vi "Datum_Image_Calibration.vi"(3 "Mode":T8=enum."Run VI", 5 "Traverse line In":T5={"Start X"=-1250.0, "Start Y"=-250.0, "Start Z"=180.0, "End X"=0.0, "End Y"=0.0, "End Z"=0.0, "No. of pts."=6, "Spacing"=enum."Linear", "Filename"=path "C:/Enflo_Data_Local/2015/EnFlo_Tunnel/Paul_Hayden/Calibrations/Cal_06-2015/Datum_Block_1.xls", "Tunnel Speed"=0.0, "Averaging time (min)"=0.01, "Extra Commands"="", "Carrier_1 Q (l/min)"=nan, "Carrier_2 Q (l/min)"=nan, "Trace Gas Concentration (%)"=nan, "Specific Arguments"="Datum_Image_Calibration.vi  ", "Comments"="", "Row No"=0, "Row Type Selector"=enum."Run VI Named:", "Completion time"="12:51  12-06-2015", "Row Duration (mins)"=0.11291999999999999, "No. of Valid pts."=6, "Meas Setup File"="Trav_Cam_Picture.xls"} {"Carrier_2 Q (l/min)" format="%#.2f"; "Row Duration (mins)" format="%#.1f"; "Row No" min=0; "Trace Gas Concentration (%)" min=0.0 format="%#_4f"; "Carrier_1 Q (l/min)" format="%#.2f"; "Tunnel Speed" format="%#.2f"; "Start X" format="%#.2f"; "Start Y" format="%#.2f"; "Start Z" format="%#.2f"; "End X" format="%#.2f"; "End Y" format="%#.2f"; "End Z" format="%#.2f"; "Averaging time (min)" min=0.0 format="%#.2f"}) -> (0 "Error Message":string, 1 "Status":T4, 2 "Traverse line Out":T5 {"Carrier_2 Q (l/min)" format="%#.2f"; "Row Duration (mins)" format="%#.1f"; "Row No" min=0; "Trace Gas Concentration (%)" min=0.0 format="%#_4f"; "Carrier_1 Q (l/min)" format="%#.2f"; "Tunnel Speed" format="%#.2f"; "Start X" format="%#.2f"; "Start Y" format="%#.2f"; "Start Z" format="%#.2f"; "End X" format="%#.2f"; "End Y" format="%#.2f"; "End Z" format="%#.2f"; "Averaging time (min)" min=0.0 format="%#.2f"})   [LabVIEW 2014]
uses:
  Gen Trav/Multi_Run_Status.ctl
  <vilib>/Analysis/NI_AALBase.lvlib
  <vilib>/Analysis/baseanly.llb/Mean (DBL).vi
  Utilities/Image acquisition and processing/Feature detection/Typedefs/Theta range.ctl
  Gen Trav/Spacing.ctl
  Gen Trav/Traverse_cluster.ctl
  Controls/User_Specific_mode.ctl
  Controls/Multi_run_mode.ctl
  <vilib>/userdefined/High Color/IMAQdx.ctl
  Utilities/Image acquisition and processing/Feature detection/Typedefs/ROI bounds.ctl
panel:
  in  "Theta range (deg)":T1={"theta max (deg)"=5.0, "theta min (deg)"=-5.0}
  in  "ROI to crop (pixels)":T2={"Xmax"=2147483647, "Ymax"=2147483647, "Xmin"=0, "Ymin"=160}
  out "Scale":dbl[](graph)
  out "Angle":dbl[](graph)
  out "Displacments":sgl[][](array[numeric])
  in  "Interface name":T3="cam2"
  in  "VideoMode":u32=9
  in  "Averaging time (s) (from end)":dbl=1.0
  in  "Duration (s)":dbl=10.0
  in  "FPS":u32=30
  in  "Video codec":string="Microsoft Video 1"
  # "X           Y            Z"
  # "Start"
  # "End"
  # "X           Y            Z"
  # "Start"
  # "End"
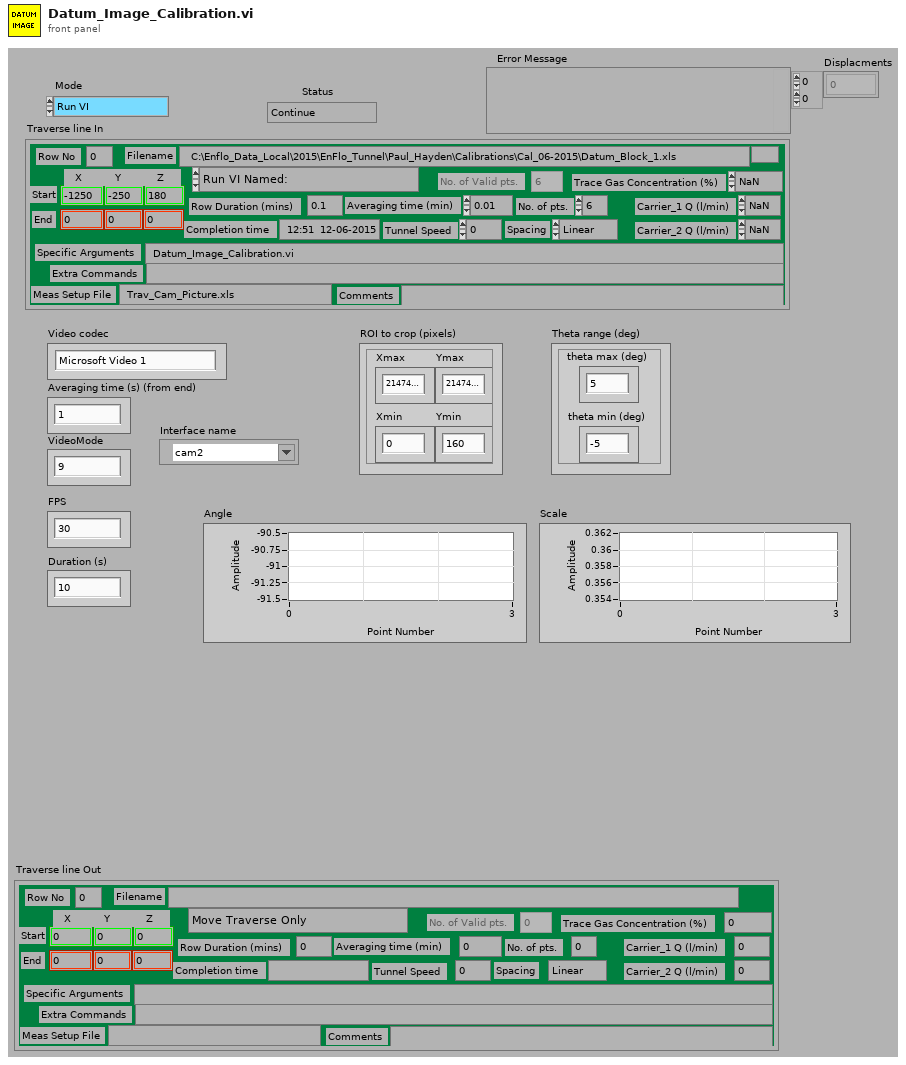
[diagram p1: front panel]
types:
  T1 = typedef "Theta range.ctl" = cluster{"theta max (deg)":dbl, "theta min (deg)":dbl}
  T2 = typedef "ROI bounds.ctl" = cluster{"Xmax":i32, "Ymax":i32, "Xmin":i32, "Ymin":i32}
  T3 = typedef "IMAQdx.ctl" = refnum<k21>
  T4 = typedef "Multi_Run_Status.ctl" = enum16{"Continue", "Jump to Next Point", "Jump to Next Row", "Jump To Fall Back", "Terminate Run"}
  T5 = typedef "Traverse_cluster.ctl" = cluster{"Start X":sgl, "Start Y":sgl, "Start Z":sgl, "End X":sgl, "End Y":sgl, "End Z":sgl, "No. of pts.":i32, "Spacing":T6, "Filename":path, "Tunnel Speed":dbl, "Averaging time (min)":dbl, "Extra Commands":string, "Carrier_1 Q (l/min)":dbl, "Carrier_2 Q (l/min)":dbl, "Trace Gas Concentration (%)":dbl, "Specific Arguments":string, "Comments":string, "Row No":i32, "Row Type Selector":T7, "Completion time":string, "Row Duration (mins)":dbl, "No. of Valid pts.":i32, "Meas Setup File":string}
  T6 = typedef "Spacing.ctl" = enum16{"Linear", "Log", "Gauss", "Specified", "N/A"}
  T7 = typedef "Multi_run_mode.ctl" = enum16{"Move Traverse Only", "Set Tunnel Speed Only", "Set Source Only", "Set Measurement Conditions", "Single Measurement", "Vertical Profile", "Lateral Profile", "Longitudinal Profile", "Explore Volume", "Multi-Axis Profile", "Auto Calibrate", "Meas Fast FID Bkgnd", "Check Beam Power", "Scanning Valve Measurement", "Run VI Named:", "Set ADAM Ch", "Wait (minutes)", "Send Message", "Synchronize With:", "Fall Back to this Row", "Turn Off Row Repeating", "Blank Row", "Traverse 3D Volume"}
  T8 = typedef "User_Specific_mode.ctl" = enum16{"Check VI only", "Run VI"}
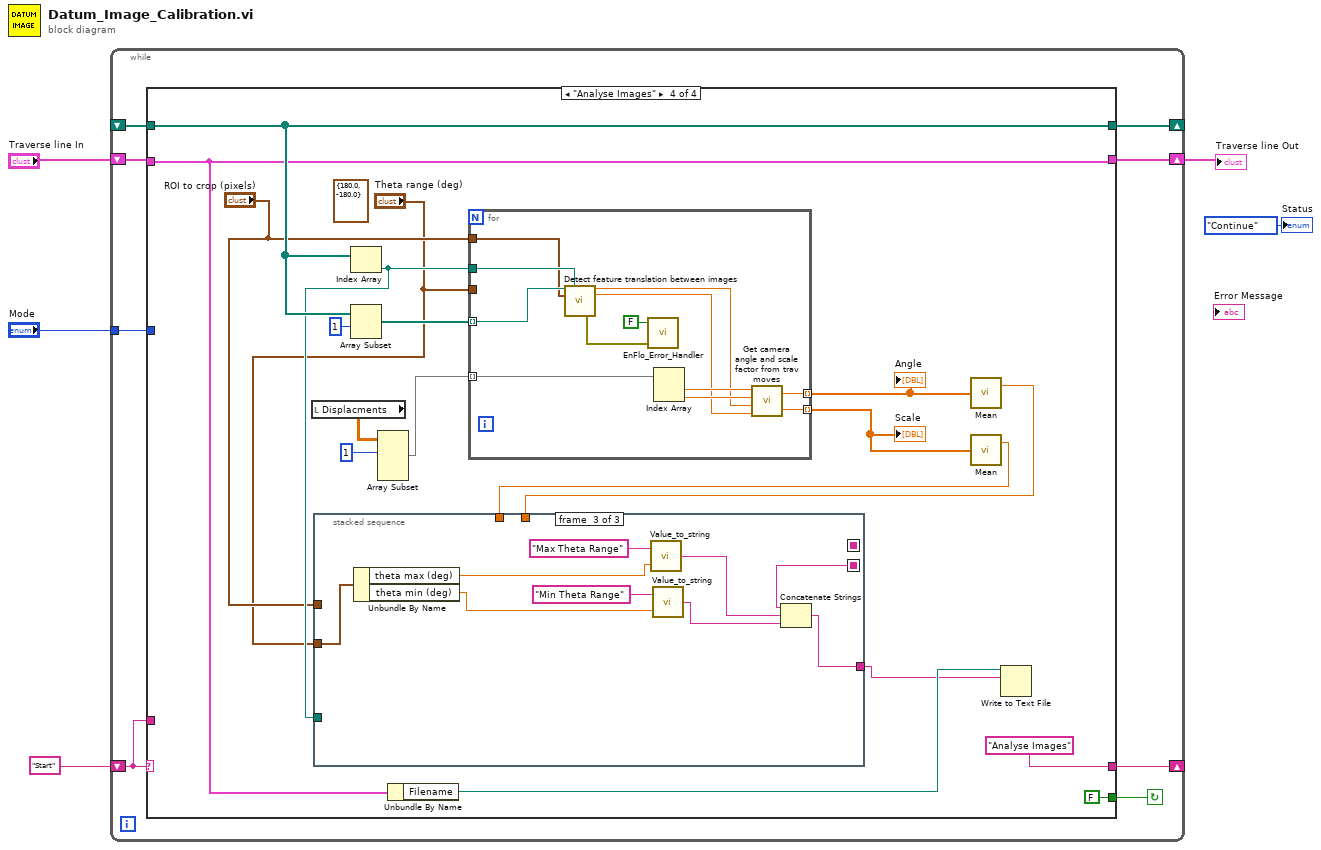
[diagram p0: block diagram]
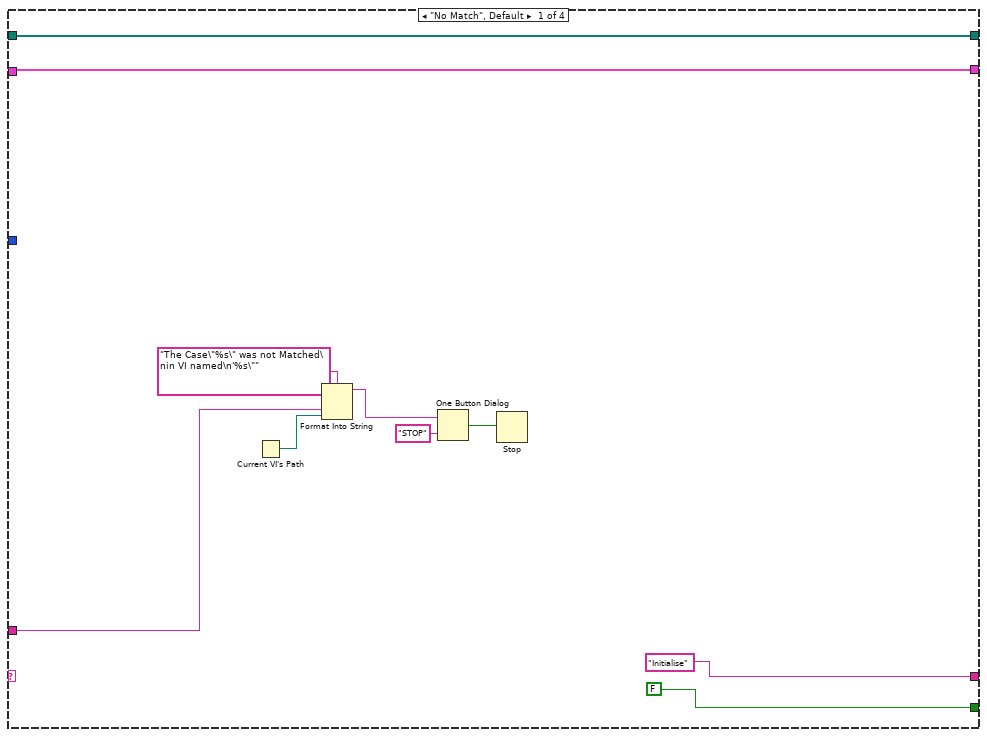
[diagram p2: hidden frame]
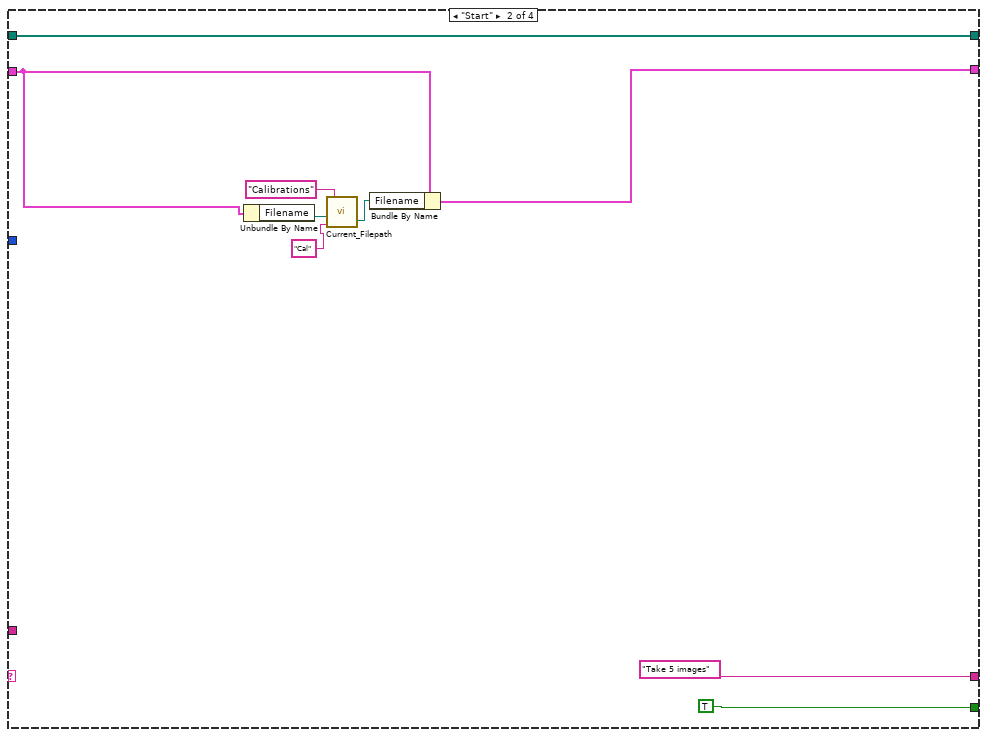
[diagram p3: hidden frame]
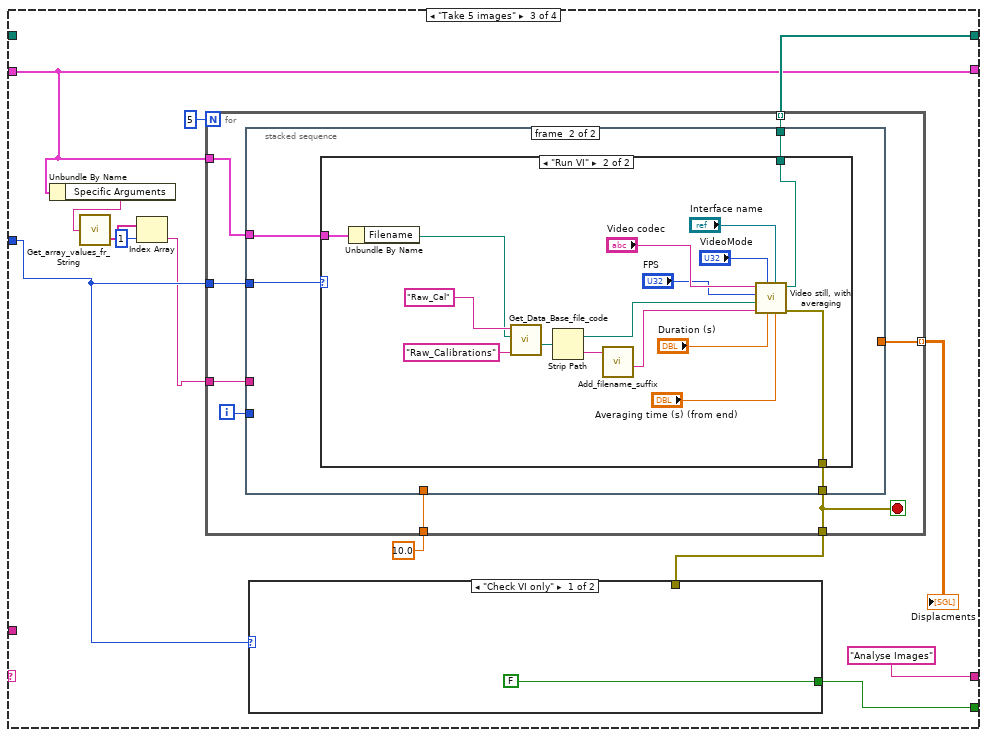
[diagram p4: hidden frame]
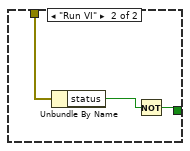
[diagram p5: hidden frame]
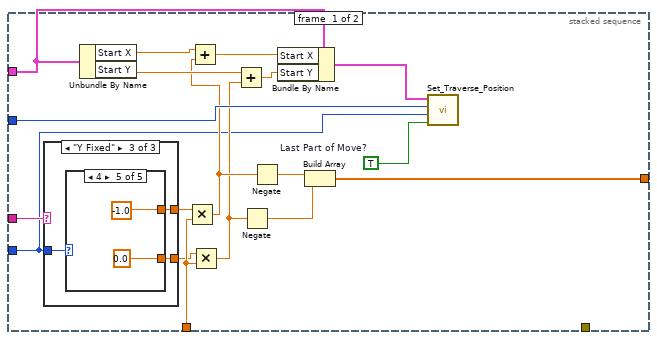
[diagram p6: hidden frame]
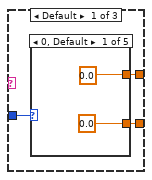
[diagram p7: hidden frame]
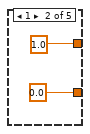
[diagram p8: hidden frame]
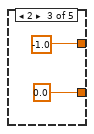
[diagram p9: hidden frame]
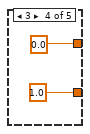
[diagram p10: hidden frame]
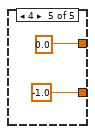
[diagram p11: hidden frame]
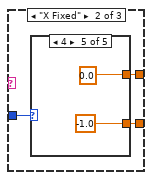
[diagram p12: hidden frame]
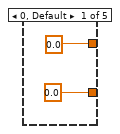
[diagram p13: hidden frame]
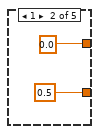
[diagram p14: hidden frame]
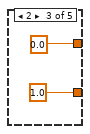
[diagram p15: hidden frame]
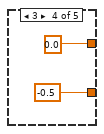
[diagram p16: hidden frame]
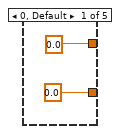
[diagram p17: hidden frame]
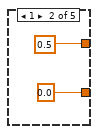
[diagram p18: hidden frame]
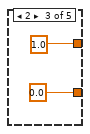
[diagram p19: hidden frame]
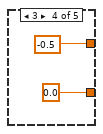
[diagram p20: hidden frame]
diagram:
  n1 = while {
    shift-left: "Start" -> [w11]
    shift-right: [w12] -> _
    tunnel: "Mode" -> [w10]
    shift-right: [w8] -> w1
    shift-left: "Traverse line In" -> [w9]
    shift-right: [w7] -> _
    shift-left: _ -> [w6]
    stop <- w13 continue-if-true
    n2 = case shown="\"Analyse Images\"" w11 {
      tunnel: [FALSE TRUE w40 FALSE] -> w13
      tunnel: ["Initialise" "Take 5 images" "Analyse Images" "Analyse Images"] -> w12
      tunnel: w11 -> [w18 _ _ _]
      tunnel: w10 -> [_ _ w41 _]
      tunnel: w9 -> [w15 w27 w37 w146]
      tunnel: [w15 w26 w37 w146] -> w8
      tunnel: [w14 w25 w42 w152] -> w7
      tunnel: w6 -> [w14 w25 _ w152]
      frame "No Match", Default {
        n3 = Current VI's Path() -> (path=w17:path)
        n4 = Format Into String(format string="The Case\"%s\" was not Matched\nin VI named\n'%s\"" ("Format String"), w18, w17) -> (resulting string=w21:string)  [unwired: 2 in, 1 out]
        n5 = One Button Dialog(message=w21, button name ("OK")="STOP") -> (true=w19:bool)
        n6 = Stop(stop? (T)=w19) -> ()
      }
      frame "Start" {
        n7 = Unbundle By Name(w27) -> ("Filename"=w29:path)
        n8 = call "Current_Filepath.vi"("Short_Name"="Cal" ("Data Type"), "Filename in"=w29, "Data Type"="Calibrations") -> ("Filename Out"=w24:path)  [unwired: 1 in, 1 out]
        n9 = Bundle By Name(cluster=w27, "Filename"=w24) -> (w26:T5)
      }
      frame "Take 5 images" {
        n10 = Unbundle By Name(w37) -> ("Specific Arguments"=w36:string)
        n11 = call "Get_array_values_fr_String.vi"("String Value"=w36) -> ("String array"=w35:string[])  [unwired: 1 out]
        n12 = Index Array(array=w35, index=1) -> (element=w33:string)
        n13 = for {
          N: 5 -> [_]
          tunnel: w37 -> [w57]
          tunnel: w41 -> [w56]
          tunnel: sgl 10.0 ("y") -> [w54]
          tunnel: [w53] -> w42 mode=indexing
          tunnel: [w52] -> w39
          tunnel: [w51] -> w38 mode=indexing
          tunnel: w33 -> [w50]
          i -> [w55]
          stop <- w52 stop-if-true
          n14 = stacked-sequence {
            tunnel: w57 -> [w67 w118]
            tunnel: w56 -> [w75 w117]
            tunnel: w55 -> [w59 _]
            tunnel: w54 -> [w72 _]
            tunnel: [_ w116] -> w53
            tunnel: [_ w115] -> w52
            tunnel: [w63 _] -> w51
            tunnel: w50 -> [w60 _]
            frame #0 {
              w58 = TRUE  # Last Part of Move?
              n15 = case shown="\"Y Fixed\"" w60 {
                tunnel: w59 -> [w78 w91 w104]
                tunnel: [w77 w90 w103] -> w73
                tunnel: [w76 w89 w102] -> w71
                frame Default {
                  n16 = case shown="0, Default" w78 {
                    tunnel: [sgl 0.0 ("Start Y") sgl 1.0 ("Start Y") sgl -1.0 ("Start Y") sgl 0.0 ("Start Y") sgl 0.0 ("Start Y")] -> w77
                    tunnel: [sgl 0.0 ("Start Y") sgl 0.0 ("Start Y") sgl 0.0 ("Start Y") sgl 1.0 ("Start Y") sgl -1.0 ("Start Y")] -> w76
                    frame 0, Default {
                    }
                    frame 1 {
                    }
                    frame 2 {
                    }
                    frame 3 {
                    }
                    frame 4 {
                    }
                  }
                }
                frame "X Fixed" {
                  n17 = case shown="4" w91 {
                    tunnel: [sgl 0.0 ("Start Y") sgl 0.0 ("Start Y") sgl 0.0 ("Start Y") sgl 0.0 ("Start Y") sgl 0.0 ("Start Y")] -> w90
                    tunnel: [sgl 0.0 ("Start Y") sgl 0.5 ("Start Y") sgl 1.0 ("Start Y") sgl -0.5 ("Start Y") sgl -1.0 ("Start Y")] -> w89
                    frame 0, Default {
                    }
                    frame 1 {
                    }
                    frame 2 {
                    }
                    frame 3 {
                    }
                    frame 4 {
                    }
                  }
                }
                frame "Y Fixed" {
                  n18 = case shown="4" w104 {
                    tunnel: [sgl 0.0 ("Start Y") sgl 0.5 ("Start Y") sgl 1.0 ("Start Y") sgl -0.5 ("Start Y") sgl -1.0 ("Start Y")] -> w103
                    tunnel: [sgl 0.0 ("Start Y") sgl 0.0 ("Start Y") sgl 0.0 ("Start Y") sgl 0.0 ("Start Y") sgl 0.0 ("Start Y")] -> w102
                    frame 0, Default {
                    }
                    frame 1 {
                    }
                    frame 2 {
                    }
                    frame 3 {
                    }
                    frame 4 {
                    }
                  }
                }
              }
              n19 = Unbundle By Name(w67) -> ("Start X"=w74:sgl, "Start Y"=w70:sgl)
              n20 = Multiply(x=w73, y=w72) -> (x*y=w65:sgl)
              n21 = Add(x=w74, y=w65) -> (x+y=w66:sgl)
              n22 = Multiply(x=w71, y=w72) -> (x*y=w64:sgl)
              n23 = Add(x=w70, y=w64) -> (x+y=w69:sgl)
              n24 = Negate(x=w64) -> (-x=w61:sgl)
              n25 = Negate(x=w65) -> (-x=w62:sgl)
              n26 = Bundle By Name(cluster=w67, "Start X"=w66, "Start Y"=w69) -> (w68:T5)
              n27 = Build Array(w62, w61) -> (w63:sgl[])
              n28 = call "Set_Traverse_Position.vi"("Last Part of Move?"=w58, "Currently on Point"=w59, "Simulate/Run"=w75, "Traverse line"=w68) -> ()  [unwired: 2 in, 1 out]
            }
            frame #1 {
              n29 = case shown="\"Run VI\"" w117 {
                tunnel: w118 -> [_ w128]
                tunnel: [path "" ("stripped path") w121] -> w116
                tunnel: [errorcluster {"status"=FALSE, "code"=0, "source"=""} ("Error Out") w123] -> w115
                frame "Check VI only" {
                }
                frame "Run VI" {
                  n30 = Unbundle By Name(w128) -> ("Filename"=w125:path)
                  n31 = call "Get_Data_Base_file_code.vi"("Data Type"="Raw_Calibrations", "Results Filename"=w125, "Short_Name"="Raw_Cal" ("Data Type")) -> ("Raw Data File Name"=w122:path)  [unwired: 1 in, 3 out]
                  n32 = Strip Path(path=w122) -> (stripped path=w124:path, name=w127:string)
                  n33 = call "Add_filename_suffix.vi"("Filename"=w127) -> ("Base name"=w126:string)  [unwired: 1 in, 3 out]
                  n34 = call "Video still, with averaging.vi"("Averaging time (s) (from end)"="Averaging time (s) (from end)", "Interface name"="Interface name", "Duration (s)"="Duration (s)", "VideoMode"="VideoMode", "Image name"=w126, "Image directory path"=w124, "FPS"="FPS", "Video codec"="Video codec") -> ("Error Out"=w123:errorcluster, "Image File"=w121:path)  [unwired: 2 in]
                }
              }
            }
          }
        }
        "Displacments" <- w38
        n35 = case shown="\"Check VI only\"" w41 {
          tunnel: [FALSE w48] -> w40
          tunnel: w39 -> [_ w49]
          frame "Check VI only" {
          }
          frame "Run VI" {
            n36 = Unbundle By Name(w49) -> ("status"=w47:bool)
            n37 = Not(x=w47) -> (.not. x?=w48:bool)
          }
        }
      }
      frame "Analyse Images" {
        (unwired) T1 {"theta max (deg)"=180.0, "theta min (deg)"=-180.0} ("Theta range (deg)")
        n38 = local read "Displacments"() -> (w150:sgl[][])
        n39 = Index Array(array=w152) -> (element=w143:path)  [unwired: 1 in]
        n40 = Array Subset(array=w152, index=1) -> (w148:path[])  [unwired: 1 in]
        n41 = Array Subset(array=w150, index (row)=1 ("index")) -> (w149:sgl[][])  [unwired: 3 in]
        n42 = Unbundle By Name(w146) -> ("Filename"=w141:path)
        n43 = for {
          tunnel: w149 -> [w202] mode=indexing
          tunnel: w143 -> [w197]
          tunnel: w148 -> [w196] mode=indexing
          tunnel: [w199] -> w145 mode=indexing
          tunnel: [w198] -> w144 mode=indexing
          tunnel: "ROI to crop (pixels)" -> [w195]
          tunnel: "Theta range (deg)" -> [_]
          n44 = call "Detect feature translation between images.vi"("Test image file path"=w196, "Reference image file path"=w197, "ROI to crop (pixels)"=w195) -> ("dx (pix)"=w194:dbl, "dy (pix)"=w193:dbl, "Error out"=w191:errorcluster)  [unwired: 8 in, 2 out]
          n45 = call "EnFlo_Error_Handler.vi"("error in (no error)"=w191, "Dialog Box (T)"=FALSE) -> ()  [unwired: 1 in, 3 out]
          n46 = Index Array(array=w202) -> (element #1=w201:sgl, element #2=w200:sgl)  [unwired: 2 in]
          n47 = call "Get camera angle and scale factor from trav moves.vi"("dy (pix)"=w193, "dx (pix)"=w194, "dy (mm)"=w200, "dx (mm)"=w201) -> ("scale factor (mm / pixel)"=w198:dbl, "camera angle, ccw+ rel. to trav. (deg)"=w199:dbl)
        }
        "Angle" <- w145
        "Scale" <- w144
        n48 = call-poly <vilib>:"Mean.vi"("X"=w145) -> ("mean"=w140:dbl)  [unwired: 1 out]
        n49 = call-poly <vilib>:"Mean.vi"("X"=w144) -> ("mean"=w142:dbl)  [unwired: 1 out]
        n50 = stacked-sequence {
          seq-local: [w156 _ _] -> [_ w169 _]
          seq-local: [_ w167 _] -> [_ _ w182]
          tunnel: w143 -> [w163 _ _]
          tunnel: w140 -> [w157 _ _]
          tunnel: w142 -> [w155 _ _]
          tunnel: "ROI to crop (pixels)" -> [_ w178 _]
          tunnel: [_ _ w184] -> w138
          tunnel: "Theta range (deg)" -> [_ _ w183]
          frame #0 {
            n51 = call "Path_2_String.vi"("Real Path"=w163) -> ("Path String"=w164:string)
            n52 = call "Value_to_string.vi"("Value"=w157, "Label for value"="Camera Angle") -> ("Output string"=w159:string)  [unwired: 1 in]
            n53 = call "Date_and_Time_to_string.vi"() -> ("Date and time (spreadsheet)"=w158:string)
            n54 = call "Value_to_string.vi"("Value"=w155, "Label for value"="scale factor (mm / pixel)") -> ("Output string"=w160:string)  [unwired: 1 in]
            n55 = call "Characters_to_string.vi"("Characters to write"=w164, "Label for characters"="Datum Image Filename") -> ("Output string"=w161:string)
            n56 = Concatenate Strings(w158, w159, w160, w161) -> (w156:string)
          }
          frame #1 {
            n57 = Unbundle By Name(w178) -> ("Xmax"=w174:i32, "Xmin"=w175:i32, "Ymax"=w176:i32, "Ymin"=w177:i32)
            n58 = call "Value_to_string.vi"("Value"=w176, "Label for value"="ROI Crop Ymax (pixels)" ("Label for characters")) -> ("Output string"=w171:string)  [unwired: 1 in]
            n59 = call "Value_to_string.vi"("Value"=w174, "Label for value"="ROI Crop Xmax (pixels)" ("Label for characters")) -> ("Output string"=w173:string)  [unwired: 1 in]
            n60 = call "Value_to_string.vi"("Value"=w177, "Label for value"="ROI Crop Ymin (pixels)" ("Label for characters")) -> ("Output string"=w170:string)  [unwired: 1 in]
            n61 = call "Value_to_string.vi"("Value"=w175, "Label for value"="ROI Crop Xmin (pixels)" ("Label for characters")) -> ("Output string"=w172:string)  [unwired: 1 in]
            n62 = Concatenate Strings(w169, w173, w172, w171, w170) -> (w167:string)
          }
          frame #2 {
            n63 = Unbundle By Name(w183) -> ("theta max (deg)"=w187:dbl, "theta min (deg)"=w188:dbl)
            n64 = call "Value_to_string.vi"("Value"=w187, "Label for value"="Max Theta Range" ("Label for characters")) -> ("Output string"=w186:string)  [unwired: 1 in]
            n65 = call "Value_to_string.vi"("Value"=w188, "Label for value"="Min Theta Range" ("Label for characters")) -> ("Output string"=w185:string)  [unwired: 1 in]
            n66 = Concatenate Strings(w182, w186, w185) -> (w184:string)
          }
        }
        n67 = Write to Text File(file (use dialog)=w141, text=w138) -> ()  [unwired: 2 in, 3 out]
      }
    }
  }
  "Traverse line Out" <- w1
  "Status" <- Multi_Run_Status."Continue" ("Status")
